vi "Target - REF - Working2.vi"() -> ()   [LabVIEW 2015]
doc: "This VI first configures the sample clock on the module and starts it. Then it acquires single point data from four channels. In order for the loop rate to be synchronized with the module's clock, the data is pipelined before it is written it to a DMA FIFO so it can be transfered to the host."
uses:
  <vilib>/LabVIEW Targets/FPGA/cRIO/shared/nicrio_ModuleControls/nicrio_cRIO-9234_DataRatesRing2.ctl
  <vilib>/rvi/Emulation/niFpgaGetClockAttributes.vi
  <vilib>/rvi/Emulation/niFpgaSctlEmulationGetInTimedLoop.vi
  <vilib>/rvi/Emulation/niFpgaEmulationReportErrorSimple.vi
  <vilib>/rvi/eio/common/nirviEmuTemplateMethod_errors.vi
  <vilib>/rvi/eio/common/nirviEmuTemplatePropertyGet_noerrors.vi
  <vilib>/rvi/Emulation/niFpgaCriticalErrorInLSC.vi
  <vilib>/rvi/eio/common/nirviEmuTemplatePropertySet_errors.vi
  <vilib>/rvi/interface/RandomDataEmulation/niFpgaRandomDataHandleErrors.vi
  <vilib>/eio/EIOMethodNode/EIOMethodNode.xnode
  <vilib>/eio/EIOPropertyNode/EIOPropertyNode.xnode
  <vilib>/eio/EIONode/EIONode.xnode
  <vilib>/rvi/DataTransferAndStorage/Container/XNode/niFpgaContainer.xnode
  <vilib>/rvi/interface/RandomDataEmulation/nirviRandomDataFpgaReadWriteTemplate.vi
  <vilib>/rvi/eio/common/nirviEmuTemplatePropertyGet_errors.vi
  <vilib>/rvi/eio/common/nirviEmuTemplatePropertySet_noerrors.vi
  GPS Timekeeper Files/FPGA Timekeeper.lvlib
panel:
  out "FPGA Timekeeper time (ns)":u64
  out "GPS status":T1(ring)
  out "FPGA Timekeeper locked":bool
  out "offset from time reference":i32
  out "antenna status":T2(ring)
  out "satellites available":u8
  out "UTC offset":i8
  out "UTC offset valid":bool
  in  "Data Rate":T3=1 items=["51.200 kS/s (NI 9234)"=1, "25.600 kS/s (NI 9234)"=2, "17.067 kS/s (NI 9234)"=3, "12.800 kS/s (NI 9234)"=4, "10.240 kS/s (NI 9234)"=5, "8.533 kS/s (NI 9234)"=6, "7.314 kS/s (NI 9234)"=7, "6.400 kS/s (NI 9234)"=8, "5.689 kS/s (NI 9234)"=9, "5.120 kS/s (NI 9234)"=10, "4.654 kS/s (NI 9234)"=11, "4.267 kS/s (NI 9234)"=12, "3.938 kS/s (NI 9234)"=13, "3.657 kS/s (NI 9234)"=14, "3.413 kS/s (NI 9234)"=15, "3.200 kS/s (NI 9234)"=16, "3.012 kS/s (NI 9234)"=17, "2.845 kS/s (NI 9234)"=18, "2.695 kS/s (NI 9234)"=19, "2.560 kS/s (NI 9234)"=20, "2.438 kS/s (NI 9234)"=21, "2.328 kS/s (NI 9234)"=22, "2.226 kS/s (NI 9234)"=23, "2.133 kS/s (NI 9234)"=24, "2.048 kS/s (NI 9234)"=25, "1.969 kS/s (NI 9234)"=26, "1.896 kS/s (NI 9234)"=27, "1.829 kS/s (NI 9234)"=28, "1.765 kS/s (NI 9234)"=29, "1.707 kS/s (NI 9234)"=30, "1.652 kS/s (NI 9234)"=31]
  out "Acq Loop Ticks":u32
  out "FPGA Error":errorcluster
  out "Module Underflow":bool
  out "DMA FIFO Full":bool
  in  "Stop":bool
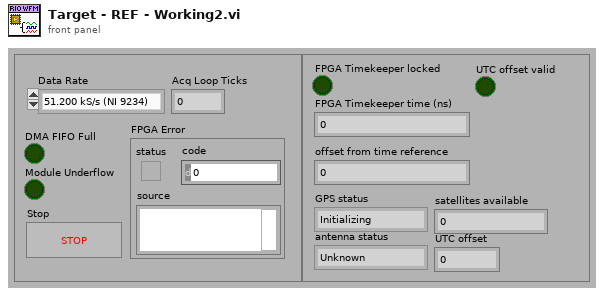
[diagram p1: front panel]
types:
  T1 = enum8{"Initializing", "Normal", "Unable to get fix"}
  T2 = enum8{"Unknown", "Normal", "Absent", "Overcurrent"}
  T3 = typedef "nicrio_cRIO-9234_DataRatesRing2.ctl" = u8
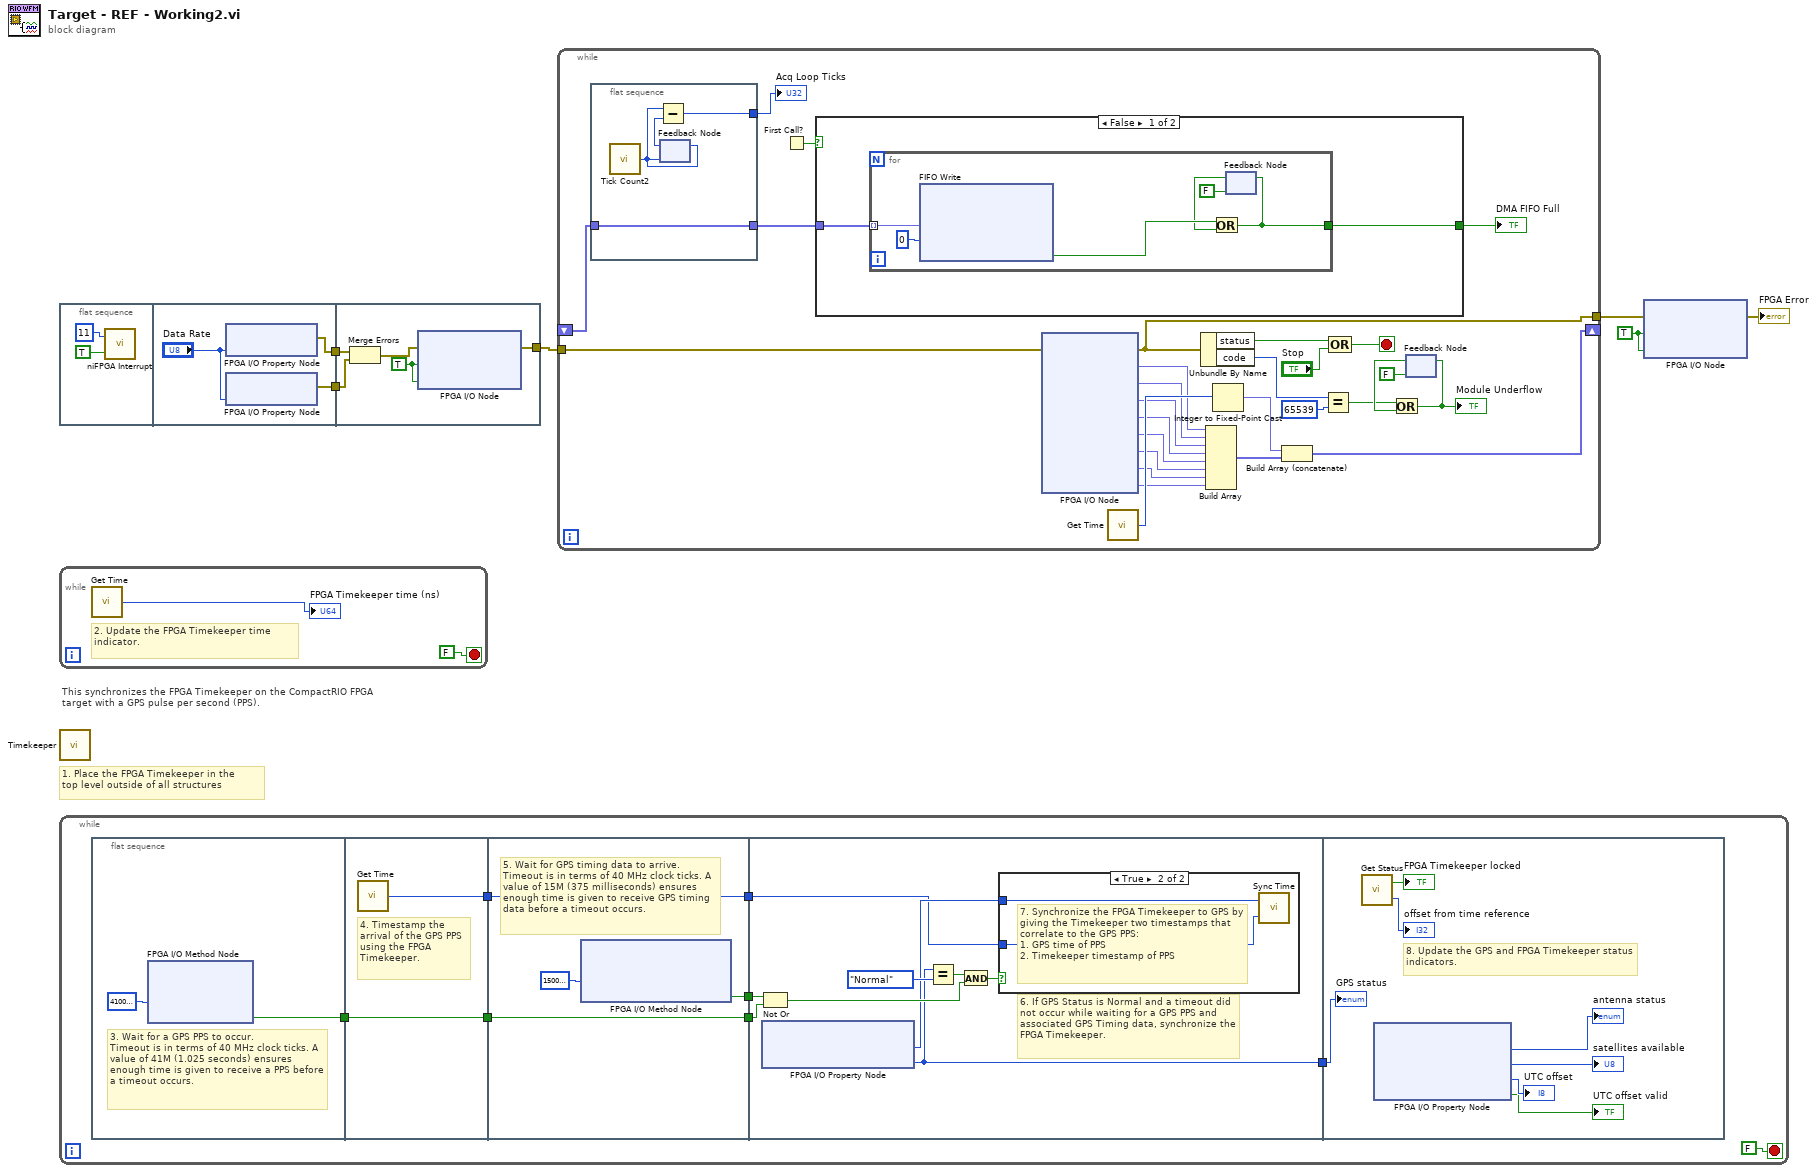
[diagram p0: block diagram]
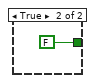
[diagram p3: hidden frame]
diagram:
  w1 = TRUE ("Mod1/Stop")
  # "This synchronizes the FPGA Timekeeper on the CompactRIO FPGA target with a GPS pulse per second (PPS)."
  # "1. Place the FPGA Timekeeper in the\ntop level outside of all structures"
  n1 = flat-sequence {
    tunnel: [w10] -> w3
    tunnel: [w9] -> w2
    tunnel: [w16] -> w6
    tunnel: w3 -> [w14]
    tunnel: w2 -> [w13]
    frame #0 {
      n2 = call <vilib>:"niFPGA Interrupt.vi"("Wait Until Cleared (F)"=TRUE ("Wait Until Cleared"), "IRQ Number (0)"=u8 11 ("IRQ Number")) -> ()  [unwired: 1 in]
    }
    frame #1 {
      n3 = xnode "FPGA I/O Property Node"("Data Rate"="Data Rate") -> ("error out"=w10:errorcluster)  [unwired: 2 in, 1 out]
      n4 = xnode "FPGA I/O Property Node"("Data Rate"="Data Rate") -> ("error out"=w9:errorcluster)  [unwired: 2 in, 1 out]
    }
    frame #2 {
      w12 = TRUE ("Mod1/Start")
      n5 = Merge Errors(w14, w13) -> (w15:errorcluster)
      n6 = xnode "FPGA I/O Node"("error in"=w15, "Mod6/Start"=w12, "Mod7/Start"=w12) -> ("error out"=w16:errorcluster)  [unwired: 2 in, 2 out]
    }
  }
  n7 = while {
    stop <- FALSE stop-if-true
    # "2. Update the FPGA Timekeeper time indicator."
    n8 = call "Get Time.vi"() -> ("time (ns)"=→"FPGA Timekeeper time (ns)":u64)  [unwired: 1 in]
  }
  n9 = call "Timekeeper.vi"() -> ()  [unwired: 12 in]
  n10 = while {
    stop <- FALSE stop-if-true
    n11 = flat-sequence {
      tunnel: [w27] -> w25
      tunnel: w25 -> [w30]
      tunnel: [w30] -> w24
      tunnel: [w29] -> w22
      tunnel: [w33] -> w26
      tunnel: w24 -> [w32]
      tunnel: [w32] -> w23
      tunnel: w22 -> [w31]
      tunnel: [w31] -> w21
      tunnel: w26 -> [w42]
      tunnel: w23 -> [w41]
      tunnel: w21 -> [w36]
      tunnel: [w35] -> w20
      tunnel: w20 -> [w52]
      frame #0 {
        # "3. Wait for a GPS PPS to occur.\nTimeout is in terms of 40 MHz clock ticks. A value of 41M (1.025 seconds) ensures enough time is given to receive a PPS before a timeout occurs."
        n12 = xnode "FPGA I/O Method Node"("Timeout"=41000000) -> ("Timed Out"=w27:bool)  [unwired: 1 in, 1 out]
      }
      frame #1 {
        # "4. Timestamp the arrival of the GPS PPS using the FPGA Timekeeper."
        n13 = call "Get Time.vi"() -> ("time (ns)"=w29:u64)  [unwired: 1 in]
      }
      frame #2 {
        # "5. Wait for GPS timing data to arrive.\nTimeout is in terms of 40 MHz clock ticks. A value of 15M (375 milliseconds) ensures enough time is given to receive GPS timing data before a timeout occurs."
        n14 = xnode "FPGA I/O Method Node"("Timeout"=15000000) -> ("Timed Out"=w33:bool)  [unwired: 1 in, 1 out]
      }
      frame #3 {
        # "6. If GPS Status is Normal and a timeout did not occur while waiting for a GPS PPS and associated GPS Timing data, synchronize the FPGA Timekeeper."
        n15 = Not Or(1:w41, 2:w42) -> (0:w39:bool)
        n16 = xnode "FPGA I/O Property Node"() -> ("PPS Timestamp (TAI)"=w37:u64, "GPS Status"=w35:T1)  [unwired: 1 in, 1 out]
        n17 = Equal?(x=w35, y=T1."Normal") -> (x = y?=w40:bool)
        n18 = And(x=w40, y=w39) -> (x .and. y?=w38:bool)
        n19 = case shown="True" w38 {
          tunnel: w37 -> [_ w45]
          tunnel: w36 -> [_ w44]
          frame False {
          }
          frame True {
            # "7. Synchronize the FPGA Timekeeper to GPS by giving the Timekeeper two timestamps that correlate to the GPS PPS:\n1. GPS time of PPS\n2. Timekeeper timestamp of PPS"
            n20 = call "Sync Time.vi"("FPGA Timekeeper time (ns)"=w44, "time reference time (ns)"=w45) -> ()
          }
        }
      }
      frame #4 {
        # "8. Update the GPS and FPGA Timekeeper status indicators."
        n21 = call "Get Status.vi"() -> ("FPGA Timekeeper locked"=→"FPGA Timekeeper locked":bool, "offset from time reference"=→"offset from time reference":i32)
        n22 = xnode "FPGA I/O Property Node"() -> ("Antenna Status"=→"antenna status":T2, "Satellites Available"=→"satellites available":u8, "UTC Offset"=→"UTC offset":i8, "UTC Offset Valid"=→"UTC offset valid":bool)  [unwired: 1 in, 1 out]
        "GPS status" <- w52
      }
    }
  }
  n23 = while {
    tunnel: [w76] -> w5
    shift-right: [w64] -> _
    shift-left: _ -> [w72]
    tunnel: w6 -> [w65]
    stop <- w79 stop-if-true
    n24 = flat-sequence {
      tunnel: [w91] -> w74
      tunnel: w72 -> [w90]
      tunnel: [w90] -> w73
      frame #0 {
        n25 = call "Tick Count2"() -> ("Tick Count(Ticks)"=w93:u32)
        n26 = feedback-in #1(w93) -> ()
        n27 = feedback #1(w93) -> (w92:u32)
        n28 = Subtract(x=w93, y=w92) -> (x-y=w91:u32)
      }
    }
    n29 = First Call?() -> (First Call?: T/F=w66:bool)
    n30 = case shown="False" w66 {
      tunnel: [w82 FALSE] -> w75
      tunnel: w73 -> [w81 _]
      frame False {
        n31 = for {
          tunnel: [w85] -> w82
          tunnel: w81 -> [w83] mode=indexing
          n32 = xnode ("FIFO Write")("Element"=w83, "Timeout"=0) -> ("Timed Out?"=w88:bool)  [unwired: 1 in, 1 out]
          n33 = feedback #2(FALSE) -> (w86:bool)
          n34 = Or(x=w88, y=w86) -> (x .or. y?=w85:bool)
          n35 = feedback-in #2(w85) -> ()
        }
      }
      frame True {
      }
    }
    "DMA FIFO Full" <- w75
    n36 = xnode "FPGA I/O Node"("error in"=w65) -> ("error out"=w76:errorcluster, "Mod6/AI0"=w60:fxp<+/-,24,4>, "Mod6/AI1"=w59:fxp<+/-,24,4>, "Mod6/AI2"=w58:fxp<+/-,24,4>, "Mod6/AI3"=w57:fxp<+/-,24,4>, "Mod7/AI0"=w56:fxp<+/-,24,4>, "Mod7/AI1"=w55:fxp<+/-,24,4>, "Mod7/AI2"=w54:fxp<+/-,24,4>, "Mod7/AI3"=w53:fxp<+/-,24,4>)  [unwired: 8 in, 8 out]
    n37 = call "Get Time.vi"() -> ("time (ns)"=w61:u64)  [unwired: 1 in]
    n38 = Unbundle By Name(w76) -> ("status"=w71:bool, "code"=w77:i32)
    n39 = Build Array(w60, w59, w58, w57, w56, w55, w54, w53) -> (w62:fxp<+/-,24,4>[])
    n40 = Integer to Fixed-Point Cast(integer=w61) -> (fixed-point=w63:fxp<+/-,64,44>)  [unwired: 1 in]
    n41 = Build Array (concatenate)(w63, w62) -> (w64:fxp<+/-,64,44>[])
    n42 = Equal?(x=w77, y=65539) -> (x = y?=w68:bool)
    n43 = Compound Arithmetic op=OR(w71, "Stop") -> (w79:bool)
    n44 = feedback #3(FALSE) -> (w70:bool)
    n45 = Or(x=w68, y=w70) -> (x .or. y?=w67:bool)
    "Module Underflow" <- w67
    n46 = feedback-in #3(w67) -> ()
    "Acq Loop Ticks" <- w74
  }
  n47 = xnode "FPGA I/O Node"("error in"=w5, "Mod6/Stop"=w1, "Mod7/Stop"=w1) -> ("error out"=→"FPGA Error":errorcluster)  [unwired: 2 in, 2 out]
